vi "Parse Capabilities for Topology.vi"(8 "error in (no error)":errorcluster, 11 "Capabilities JSON In":string) -> (0 "error out":errorcluster, 3 "Topology Info":T1[](array[typedef]))   [LabVIEW 2015, in "SLSC Switch.lvlib" / "SLSC Switch.lvclass"]
uses:
  SLSC Switch.lvclass
  Controls/JSON.ConnectionList.ctl
  Controls/JSON.ChannelList.ctl
  Controls/JSON.InitialState.ctl
  Controls/Topology.ctl
  Controls/JSON.NoMux.Topology.ctl
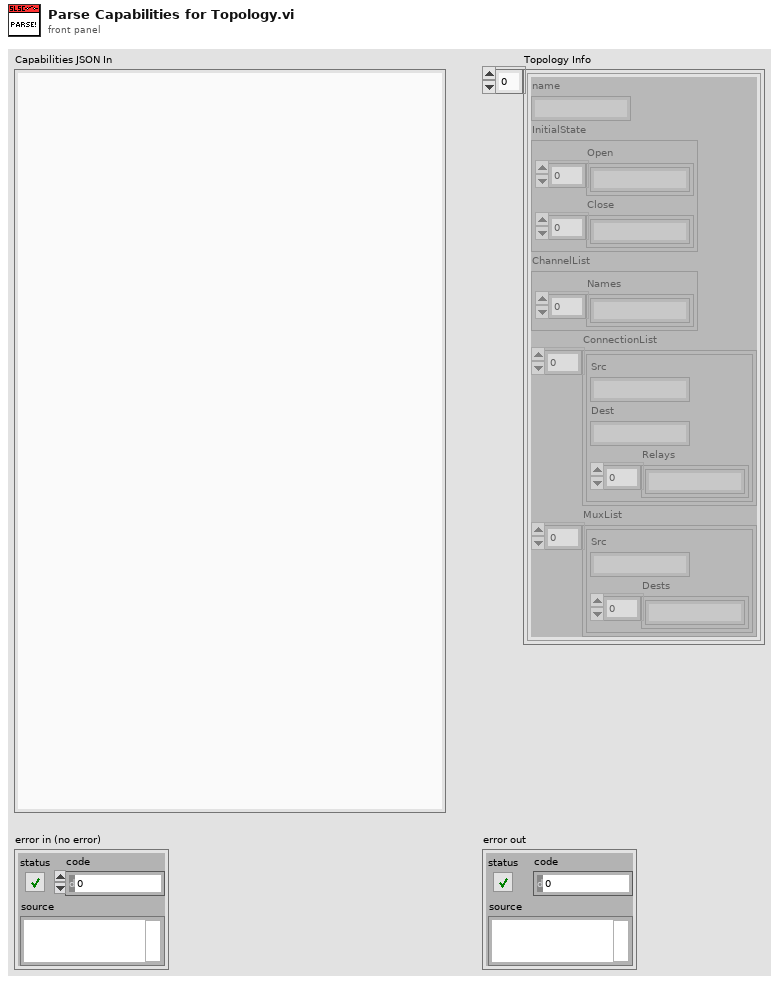
[diagram p1: front panel]
types:
  T1 = typedef "SLSC Switch.lvlib/SLSC Switch.lvclass/Topology.ctl" = cluster{"name":string, "InitialState":T2, "ChannelList":T3, "ConnectionList":T4[], "MuxList":cluster{"Src":string, "Dests":string[]}[]}
  T2 = typedef "SLSC Switch.lvlib/SLSC Switch.lvclass/JSON.InitialState.ctl" = cluster{"Open":string[], "Close":string[]}
  T3 = typedef "SLSC Switch.lvlib/SLSC Switch.lvclass/JSON.ChannelList.ctl" = cluster{"Names":string[]}
  T4 = typedef "SLSC Switch.lvlib/SLSC Switch.lvclass/JSON.ConnectionList.ctl" = cluster{"Src":string, "Dest":string, "Relays":string[]}
  T5 = typedef "SLSC Switch.lvlib/SLSC Switch.lvclass/JSON.NoMux.Topology.ctl" = cluster{"name":string, "InitialState":T2, "ChannelList":T3, "ConnectionList":T4[]}
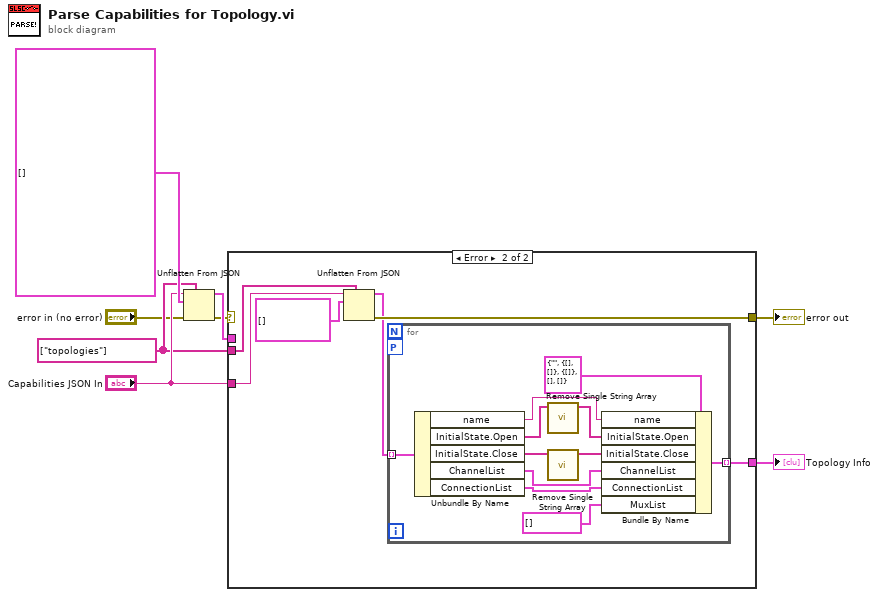
[diagram p0: block diagram]
diagram:
  w5 = string[] ["topologies"] ("path")
  n1 = Unflatten From JSON(path=w5, JSON string="Capabilities JSON In", type and defaults=T1[] [] ("Array"), error in (no error)="error in (no error)") -> (value=w4:T1[], error out=w3:errorcluster)  [unwired: 3 in]
  n2 = case shown="Error" w3 {
    selector: w3 -> [w9 _]
    tunnel: w4 -> [w10 _]
    tunnel: w5 -> [_ w16]
    tunnel: "Capabilities JSON In" -> [_ w15]
    tunnel: [w9 w13] -> w1
    tunnel: [w10 w11] -> w8
    frame No Error {
    }
    frame Error {
      n3 = Unflatten From JSON(path=w16, JSON string=w15, type and defaults=T5[] [] ("Array")) -> (value=w12:T5[], error out=w13:errorcluster)  [unwired: 4 in]
      n4 = for {
        tunnel: w12 -> [w26] mode=indexing
        tunnel: [w21] -> w11 mode=indexing
        workers-P: _ -> [_]
        n5 = Unbundle By Name(w26) -> ("name"=w25:string, "InitialState.Open"=w18:string[], "InitialState.Close"=w20:string[], "ChannelList"=w24:T3, "ConnectionList"=w23:T4[])
        n6 = call "Remove Single String Array.vi"("Close in"=w18) -> ("Close out"=w17:string[])  [unwired: 10 in]
        n7 = call "Remove Single String Array.vi"("Close in"=w20) -> ("Close out"=w19:string[])  [unwired: 10 in]
        n8 = Bundle By Name(cluster=T1 {"name"="", "InitialState"={"Open"=[], "Close"=[]}, "ChannelList"={"Names"=[]}, "ConnectionList"=[], "MuxList"=[]} ("Topology"), "name"=w25, "InitialState.Open"=w17, "InitialState.Close"=w19, "ChannelList"=w24, "ConnectionList"=w23, "MuxList"=cluster{"Src":string, "Dests":string[]}[] []) -> (w21:T1)
      }
    }
  }
  "Topology Info" <- w8
  "error out" <- w1
